vi "UTIL Open Feature File.vi"(8 "Error In":errorcluster, 10 "Testing":bool) -> (0 "Error Out":errorcluster, 3 "Feature File Refnum":refnum<file>)   [LabVIEW 2010]
doc: "This VI opens the Feature File used to write binary data related to the EMG/EEG Power and Stimulus settings. It has a Testing input (default False) that specifies the file Test.bin on LabVIEW's Temp folder, automatically overwriting an existing file without confirmation.\n\nThe default behavior is to write a specific file, named in this VI, and to request confirmation for replacement.\n\nInputs:\n Testing Boolean (default False)\n Error In\nOutputs:\n Feature File Refnum Refnum to opened Feature File\n Error Out"
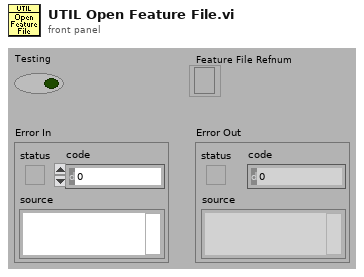
[diagram p1: front panel]
types:
  T1 = enum16{"open", "replace", "create", "open or create", "replace or create", "replace or create with confirmation"}
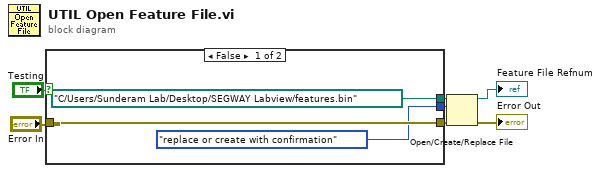
[diagram p0: block diagram]
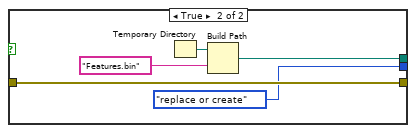
[diagram p2: hidden frame]
diagram:
  n1 = case shown="False" "Testing" {
    tunnel: "Error In" -> [w10 w13]
    tunnel: [w10 w13] -> w6
    tunnel: [path "C:/Users/Sunderam Lab/Desktop/SEGWAY Labview/features.bin" ("Filename") w12] -> w4
    tunnel: [T1."replace or create with confirmation" ("operation (0:open)") T1."replace or create" ("operation (0:open)")] -> w3
    frame False {
    }
    frame True {
      n2 = Temporary Directory() -> (w15:path)
      n3 = Build Path(base path=w15, name or relative path="Features.bin") -> (appended path=w12:path)
    }
  }
  n4 = Open/Create/Replace File(file path (use dialog)=w4, error in=w6, operation (0:open)=w3) -> (refnum out=→"Feature File Refnum":refnum<file>, error out=→"Error Out":errorcluster)  [unwired: 3 in, 1 out]
